vi "Tektronix_Config.vi"(0 "Oscilloscope-Change":bool=TRUE, 1 "Vertical Coupling (1: DC)":i32(ring)=1 items=["AC", "DC", "Ground"], 2 "TestIndex":i32, 3 "Probe Attenuation (10: 10X)":i32(ring)=1 items=["1"=1, "10"=10, "20"=20, "50"=50, "100"=100, "500"=500, "1000"=1000], 4 "Vertical Range (10.0 V/div)":dbl=5.0, 5 "error in (no error)":errorcluster, 6 "Vertical Offset (0.0 divs)":dbl=-1.0, 7 "Bandwidth (0: MAX Bandwidth)":i32(ring) items=["MAX Bandwidth", "Unlimited"], 8 "Channel (0: Channel 1)":i32(ring) items=["Channel 1", "Channel 2", "Channel 3", "Channel 4", "Math", "Reference A", "Reference B", "Reference C", "Reference D"], 10 "Enable Channel (True)":bool=TRUE, 11 "Timebase (0.0005 s)":dbl=0.00025, 12 "Trigger Level (0.0 V)":dbl=10.0, 15 "Trigger Mode (0: Auto)":i32(ring) items=["Auto", "Normal"], 17 "Holdoff (0.00)":dbl format="%_3g", 18 "Trigger Slope (0: Rising)":i32(ring) items=["Rising", "Falling"]) -> (14 "VISA":refnum<visa-resource-name>, 19 "error out":errorcluster)   [LabVIEW 2015]
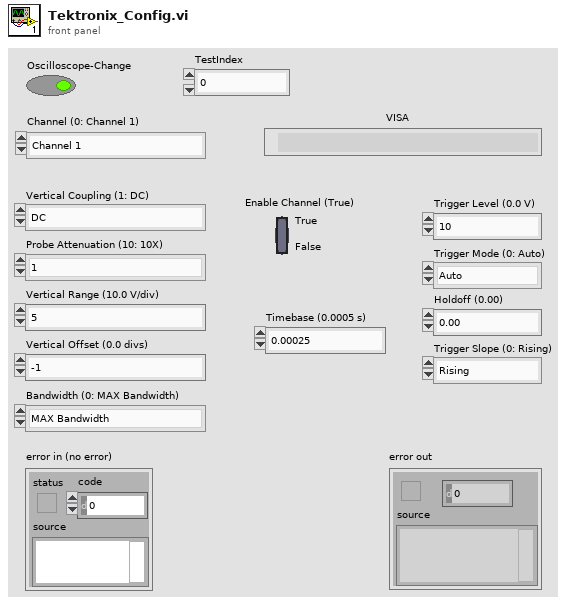
[diagram p1: front panel]
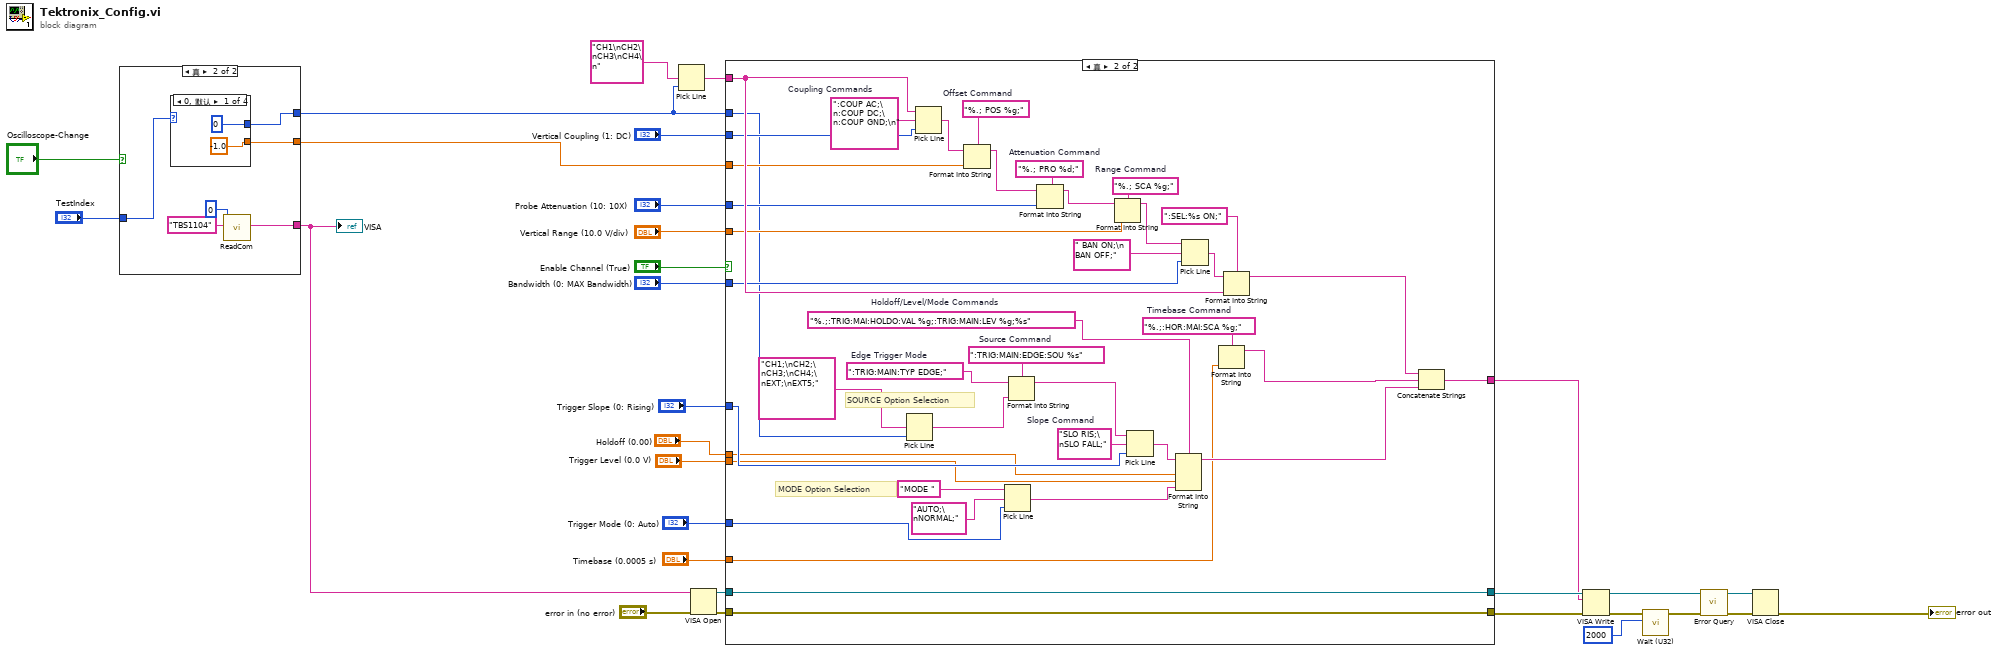
[diagram p0: block diagram]
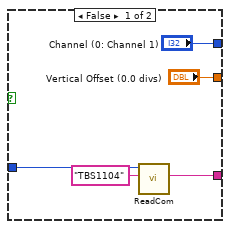
[diagram p2: hidden frame]
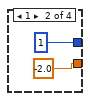
[diagram p3: hidden frame]
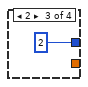
[diagram p4: hidden frame]
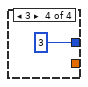
[diagram p5: hidden frame]
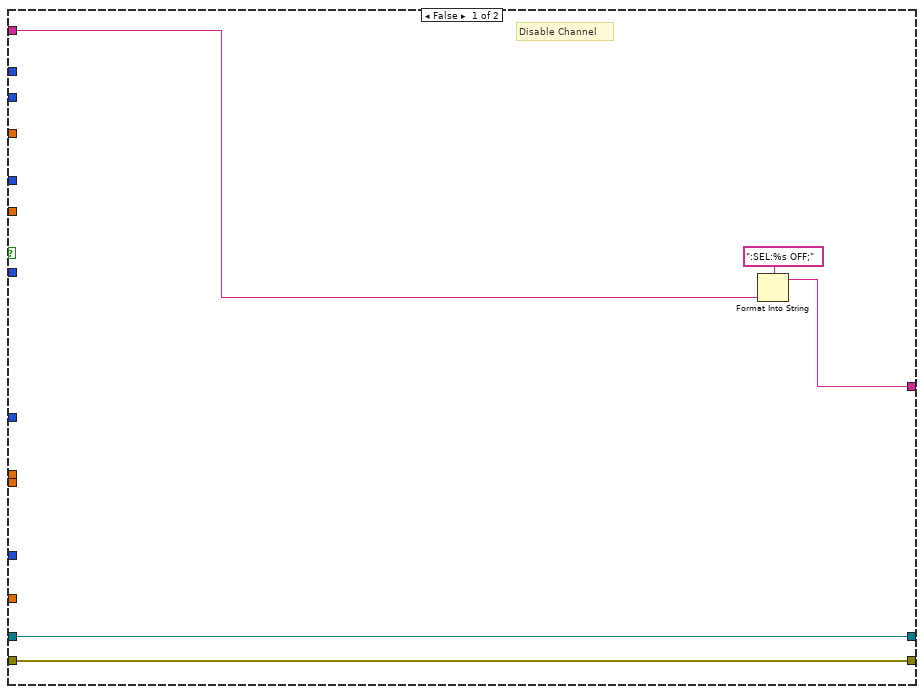
[diagram p6: hidden frame]
diagram:
  n1 = case shown="真" "Oscilloscope-Change" {
    tunnel: ["Channel (0: Channel 1)" w41] -> w14
    tunnel: ["Vertical Offset (0.0 divs)" w40] -> w13
    tunnel: "TestIndex" -> [w32 w39]
    tunnel: [w31 w37] -> w1
    frame False {
      n2 = call "ReadCom.vi"("仪器名称"="TBS1104", "MyIndex"=w32) -> ("COM"=w31:string)  [unwired: 7 in, 2 out]
    }
    frame True {
      n3 = case shown="0, 默认" w39 {
        tunnel: [0 1 2 3] -> w41
        tunnel: [-1.0 ("Vertical Offset (0.0 divs)") -2.0 ("Vertical Offset (0.0 divs)") _ _] -> w40
        frame 0, Default {
        }
        frame 1 {
        }
        frame 2 {
        }
        frame 3 {
        }
      }
      n4 = call "ReadCom.vi"("仪器名称"="TBS1104", "MyIndex"=u8 0) -> ("COM"=w37:string)  [unwired: 7 in, 2 out]
    }
  }
  "VISA" <- w1
  n5 = Pick Line(multi-line string="CH1\nCH2\nCH3\nCH4\n", line index=w14) -> (output string=w28:string)  [unwired: 1 out]
  n6 = VISA Open(error in (no error)="error in (no error)", VISA resource name=w1) -> (VISA resource name=w12:refnum<visa-resource-name>, error out=w11:errorcluster)  [unwired: 3 in]
  n7 = case shown="真" "Enable Channel (True)" {
    tunnel: w28 -> [w51 w91]
    tunnel: w14 -> [_ w64]
    tunnel: "Vertical Coupling (1: DC)" -> [_ w90]
    tunnel: w13 -> [_ w89]
    tunnel: "Probe Attenuation (10: 10X)" -> [_ w88]
    tunnel: "Vertical Range (10.0 V/div)" -> [_ w87]
    tunnel: "Bandwidth (0: MAX Bandwidth)" -> [_ w86]
    tunnel: "Trigger Slope (0: Rising)" -> [_ w63]
    tunnel: "Holdoff (0.00)" -> [_ w62]
    tunnel: "Trigger Level (0.0 V)" -> [_ w61]
    tunnel: "Trigger Mode (0: Auto)" -> [_ w60]
    tunnel: w12 -> [w49 w54]
    tunnel: [w49 w54] -> w17
    tunnel: [w48 w55] -> w16
    tunnel: w11 -> [w48 w55]
    tunnel: "Timebase (0.0005 s)" -> [_ w57]
    tunnel: [w50 w56] -> w15
    frame False {
      # "Disable Channel"
      n8 = Format Into String(format string=":SEL:%s OFF;", w51) -> (resulting string=w50:string)  [unwired: 2 in, 1 out]
    }
    frame True {
      w65 = "%.;:HOR:MAI:SCA %g;"  # Timebase Command
      w69 = "SLO RIS;\nSLO FALL;"  # Slope Command
      w68 = "%.;:TRIG:MAI:HOLDO:VAL %g;:TRIG:MAIN:LEV %g;%s"  # Holdoff/Level/Mode Commands
      w67 = ":TRIG:MAIN:TYP EDGE;"  # Edge Trigger Mode
      w66 = ":TRIG:MAIN:EDGE:SOU %s"  # Source Command
      w82 = "%.; PRO %d;"  # Attenuation Command
      w83 = "%.; SCA %g;"  # Range Command
      w84 = "%.; POS %g;"  # Offset Command
      w85 = ":COUP AC;\n:COUP DC;\n:COUP GND;\n"  # Coupling Commands
      # "MODE Option Selection"
      # "SOURCE Option Selection"
      n9 = Pick Line(multi-line string="CH1;\nCH2;\nCH3;\nCH4;\nEXT;\nEXT5;", line index=w64) -> (output string=w73:string)  [unwired: 1 out]
      n10 = Pick Line(string ("")=w91, multi-line string=w85, line index=w90) -> (output string=w81:string)
      n11 = Format Into String(format string=w84, initial string=w81, w89) -> (resulting string=w79:string)  [unwired: 1 in, 1 out]
      n12 = Pick Line(string ("")="MODE ", multi-line string="AUTO;\nNORMAL;", line index=w60) -> (output string=w76:string)
      n13 = Format Into String(format string=w66, initial string=w67, w73) -> (resulting string=w70:string)  [unwired: 1 in, 1 out]
      n14 = Format Into String(format string=w82, initial string=w79, w88) -> (resulting string=w78:string)  [unwired: 1 in, 1 out]
      n15 = Format Into String(format string=w83, initial string=w78, w87) -> (resulting string=w77:string)  [unwired: 1 in, 1 out]
      n16 = Pick Line(string ("")=w70, multi-line string=w69, line index=w63) -> (output string=w71:string)
      n17 = Format Into String(format string=w68, initial string=w71, w62, w61, w76) -> (resulting string=w58:string)  [unwired: 1 in, 1 out]
      n18 = Pick Line(string ("")=w77, multi-line string=" BAN ON;\n BAN OFF;", line index=w86) -> (output string=w92:string)
      n19 = Format Into String(format string=w65, w57) -> (resulting string=w53:string)  [unwired: 2 in, 1 out]
      n20 = Format Into String(format string=":SEL:%s ON;", initial string=w92, w91) -> (resulting string=w59:string)  [unwired: 1 in, 1 out]
      n21 = Concatenate Strings(w59, w53, w58) -> (w56:string)
    }
  }
  n22 = VISA Write(VISA resource name=w17, write buffer=w15, error in (no error)=w16) -> (VISA resource name out=w18:refnum<visa-resource-name>, error out=w3:errorcluster)  [unwired: 1 out]
  n23 = call "Wait (U32).vi"("ms"=u32 2000 ("等待时间（毫秒）"), "Error In"=w3) -> ("Error Out"=w2:errorcluster)  [unwired: 5 in]
  n24 = call "Error Query.vi"("error in (no error)"=w2, "VISA resource name"=w18) -> ("error out"=w9:errorcluster, "VISA resource name out"=w8:refnum<visa-resource-name>)  [unwired: 8 out]
  n25 = VISA Close(VISA resource name=w8, error in (no error)=w9) -> (error out=→"error out":errorcluster)
